vi "Global Stop 2.vi"() -> ()   [LabVIEW 2020]
panel:
  out "global stop 2":bool
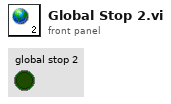
[diagram p1: front panel]
diagram:
